vi "PS_Open-Cmd-Close.vi"(3 "Error In":errorcluster, 5 "PS COM Port Ref":refnum<visa-resource-name>) -> (0 "Error Out":errorcluster)   [LabVIEW 2017]
panel:
  # "This VI exercises the Agilent E3631A \nTriple Output DC Power Supply\n\nCommunication port: RS-232, 9600 Baud,\n None Parity,  8 Bits"
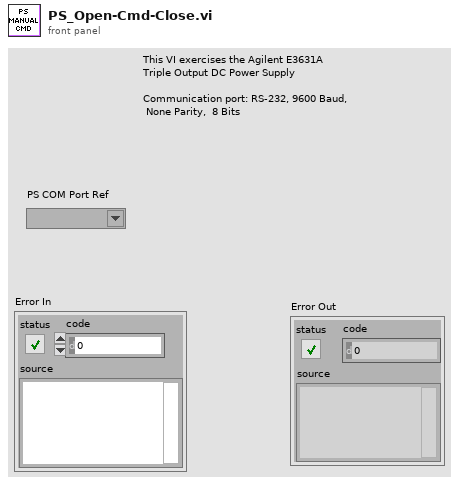
[diagram p1: front panel]
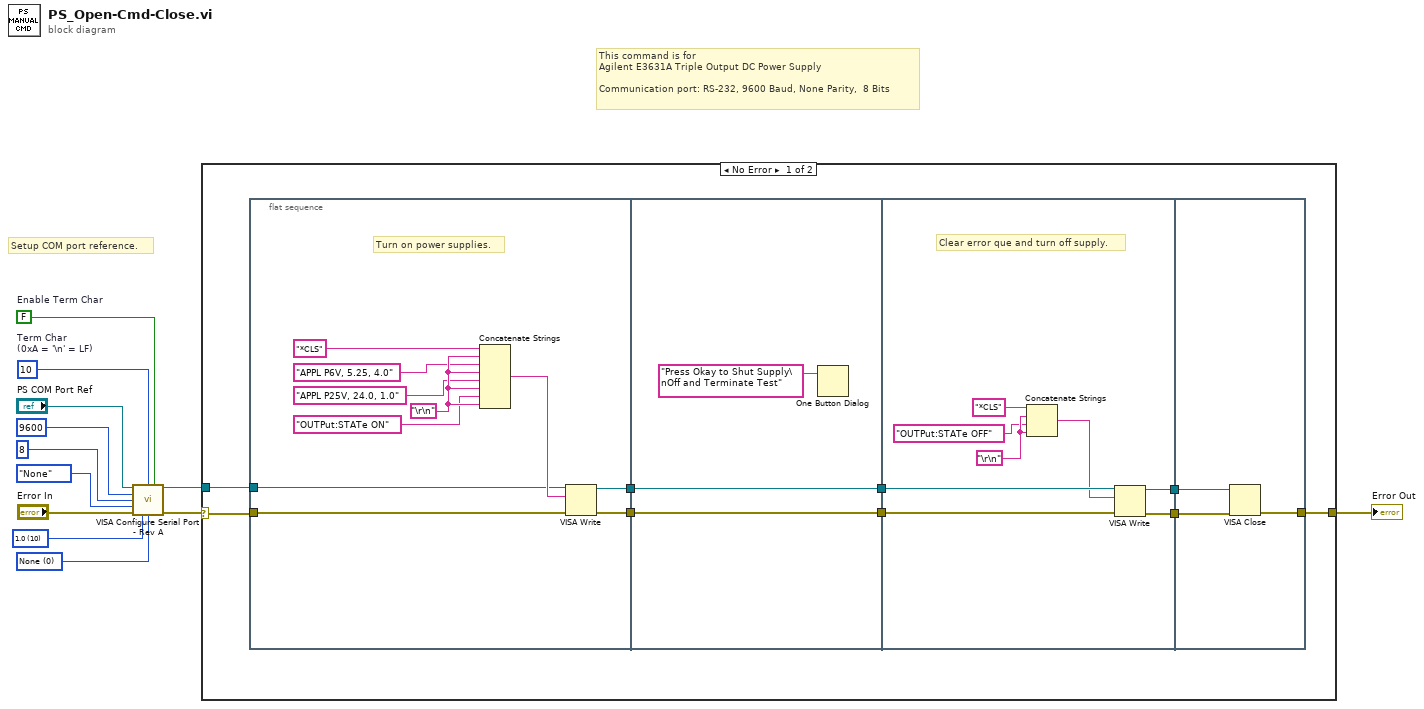
[diagram p0: block diagram]
diagram:
  w9 = u8 10  # Term Char (0xA = '\n' = LF)
  w3 = u16 0 items=["None", "XON/XOFF", "RTS/CTS", "XON/XOFF & RTS/CTS", "DTR/DSR", "XON/XOFF & DTR/DSR"] ("flow control (0:none)")
  w4 = u16 10 items=["1.0"=10, "1.5"=15, "2.0"=20] ("stop bits 4")
  w8 = FALSE  # Enable Term Char
  # "Setup COM port reference."
  # "This command is for\nAgilent E3631A Triple Output DC Power Supply\n\nCommunication port: RS-232, 9600 Baud, None Parity,  8 Bits"
  n1 = call "VISA Configure Serial Port - Rev A.vi"("VISA resource name"="PS COM Port Ref", "termination char\n(0xA = '\\n' = LF)"=w9, "Enable Termination\nChar (T)"=w8, "baud rate (9600)"=u32 9600, "data bits (8)"=u16 8 ("data bits 4"), "parity (0:none)"=enum16{"None", "Odd", "Even", "Mark", "Space"}."None" ("parity 4"), "error in (no error)"="Error In", "stop bits (10: 1 bit)"=w4, "flow control (0:none)"=w3) -> ("VISA resource name out"=w1:refnum<visa-resource-name>, "error out"=w2:errorcluster)  [unwired: 5 in]
  n2 = case shown="No Error" w2 {
    selector: w2 -> [w14 w46]
    tunnel: [w15 w46] -> w12
    tunnel: w1 -> [w13 _]
    frame No Error {
      n3 = flat-sequence {
        tunnel: [w31] -> w21
        tunnel: [w30] -> w20
        tunnel: w14 -> [w23]
        tunnel: w13 -> [w22]
        tunnel: [w33] -> w19
        tunnel: w21 -> [w33]
        tunnel: [w32] -> w18
        tunnel: w20 -> [w32]
        tunnel: w19 -> [w39]
        tunnel: w18 -> [w38]
        tunnel: [w36] -> w17
        tunnel: [w35] -> w16
        tunnel: w17 -> [w45]
        tunnel: w16 -> [w44]
        tunnel: [w43] -> w15
        frame #0 {
          w28 = "\r\n"
          # "Turn on power supplies."
          n4 = Concatenate Strings("*CLS" ("write buffer"), w28, "APPL P6V, 5.25, 4.0" ("write buffer"), w28, "APPL P25V, 24.0, 1.0" ("write buffer"), w28, "OUTPut:STATe ON" ("write buffer"), w28) -> (w24:string)
          n5 = VISA Write(VISA resource name=w22, write buffer=w24, error in (no error)=w23) -> (VISA resource name out=w30:refnum<visa-resource-name>, error out=w31:errorcluster)  [unwired: 1 out]
        }
        frame #1 {
          n6 = One Button Dialog(message="Press Okay to Shut Supply\nOff and Terminate Test") -> ()  [unwired: 1 in, 1 out]
        }
        frame #2 {
          w41 = "\r\n"
          # "Clear error que and turn off supply."
          n7 = Concatenate Strings("*CLS" ("write buffer"), w41, "OUTPut:STATe OFF" ("write buffer"), w41) -> (w37:string)
          n8 = VISA Write(VISA resource name=w38, write buffer=w37, error in (no error)=w39) -> (VISA resource name out=w36:refnum<visa-resource-name>, error out=w35:errorcluster)  [unwired: 1 out]
        }
        frame #3 {
          n9 = VISA Close(VISA resource name=w45, error in (no error)=w44) -> (error out=w43:errorcluster)
        }
      }
    }
    frame Error {
    }
  }
  "Error Out" <- w12
